vi "TCP-Send Command Receive DBL (2D).vi"(0 "PXI Address":string, 5 "Port":i32, 7 "Command":string, 9 "timeout (ms)":i32=5000, 11 "error in (no error)":errorcluster) -> (6 "data":dbl[][](array[numeric]), 10 "result":i32, 15 "error out":errorcluster)   [LabVIEW 2020]
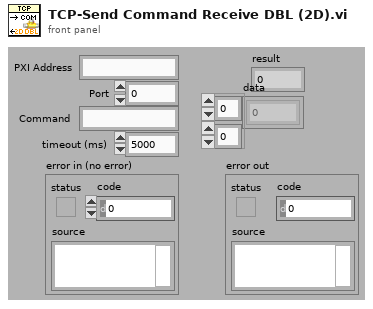
[diagram p1: front panel]
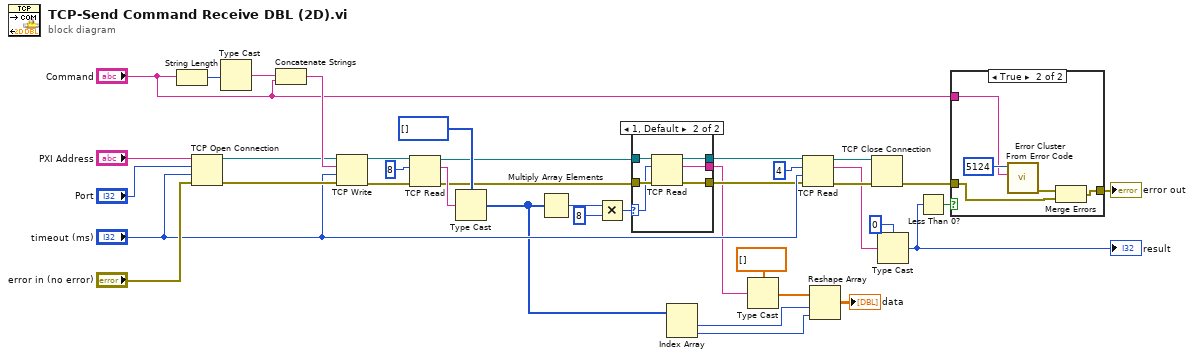
[diagram p0: block diagram]
diagram:
  n1 = String Length(string="Command") -> (length=w34:i32)
  n2 = TCP Open Connection(address="PXI Address", remote port or service name="Port", timeout ms (60000)="timeout (ms)", error in (no error)="error in (no error)") -> (connection ID=w31:refnum<k5>, error out=w32:errorcluster)  [unwired: 1 in]
  n3 = Type Cast(x=w34) -> (*(type *) &x=w33:string)  [unwired: 1 in]
  n4 = Concatenate Strings(w33, "Command") -> (w35:string)
  n5 = TCP Write(connection ID=w31, data in=w35, error in (no error)=w32, 9:"timeout (ms)") -> (connection ID out=w17:refnum<k5>, error out=w16:errorcluster)  [unwired: 1 out]
  n6 = TCP Read(connection ID=w17, bytes to read=8, error in (no error)=w16) -> (connection ID out=w4:refnum<k5>, data out=w19:string, error out=w3:errorcluster)  [unwired: 2 in]
  n7 = Type Cast(type=i32[] [], x=w19) -> (*(type *) &x=w6:i32[])
  n8 = Multiply Array Elements(1:w6) -> (0:w5:i32)
  n9 = Multiply(x=w5, y=8) -> (x*y=w2:i32)
  n10 = case shown="1, Default" w2 {
    selector: w2 -> [_ w41]
    tunnel: [_ w46] -> w11
    tunnel: [w40 w45] -> w14
    tunnel: w4 -> [w39 w44]
    tunnel: w3 -> [w40 w43]
    tunnel: [w39 w42] -> w15
    frame 0 {
    }
    frame 1, Default {
      n11 = TCP Read(connection ID=w44, bytes to read=w41, error in (no error)=w43) -> (connection ID out=w42:refnum<k5>, data out=w46:string, error out=w45:errorcluster)  [unwired: 2 in]
    }
  }
  n12 = Index Array(array=w6) -> (element #1=w9:i32, element #2=w8:i32)  [unwired: 2 in]
  n13 = Type Cast(type=dbl[] [], x=w11) -> (*(type *) &x=w10:dbl[])
  n14 = TCP Read(connection ID=w15, bytes to read=4, error in (no error)=w14, 9:"timeout (ms)") -> (connection ID out=w27:refnum<k5>, data out=w26:string, error out=w28:errorcluster)  [unwired: 1 in]
  n15 = Reshape Array(w10, w9, w8) -> (→"data":dbl[][])
  n16 = TCP Close Connection(connection ID=w27, error in (no error)=w28) -> (error out=w21:errorcluster)  [unwired: 1 in, 1 out]
  n17 = Type Cast(type=0, x=w26) -> (*(type *) &x=w24:i32)
  "result" <- w24
  n18 = Less Than 0?(x=w24) -> (x < 0?=w23:bool)
  n19 = case shown="True" w23 {
    tunnel: [w47 w49] -> w22
    tunnel: w21 -> [w47 w48]
    tunnel: "Command" -> [_ w50]
    frame False {
    }
    frame True {
      n20 = call <vilib>:"Error Cluster From Error Code.vi"("error message (\"\")"=w50, "error code (0)"=5124) -> ("error out"=w52:errorcluster)  [unwired: 7 in]
      n21 = Merge Errors(w52, w48) -> (w49:errorcluster)
    }
  }
  "error out" <- w22
